vi "Write Device_Name.vi"(8 "error in (no error)":errorcluster, 10 "Device_Name":string, 11 "Processor in":refnum<class "Processor.lvclass">) -> (0 "error out":errorcluster, 3 "Processor out":refnum<class "Processor.lvclass">)   [LabVIEW 2025, in "Processor.lvclass"]
uses:
  Processor.lvclass
  Processor.lvclass/Processor.ctl
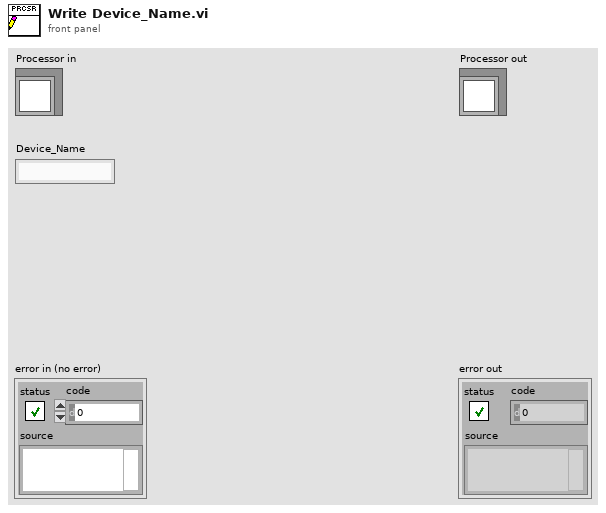
[diagram p1: front panel]
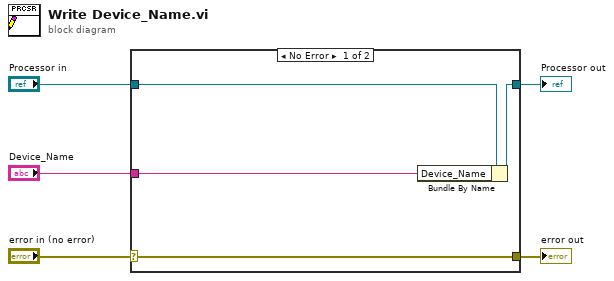
[diagram p0: block diagram]
diagram:
  n1 = case shown="No Error" "error in (no error)" {
    selector: "error in (no error)" -> [w9 w10]
    tunnel: [w9 w10] -> w4
    tunnel: [w7 w11] -> w2
    tunnel: "Processor in" -> [w8 w11]
    tunnel: "Device_Name" -> [w6 _]
    frame No Error {
      n2 = Bundle By Name(cluster=w8, "Device_Name"=w6) -> (w7:refnum<class "Processor.lvclass">)
    }
    frame Error {
    }
  }
  "error out" <- w4
  "Processor out" <- w2
